vi "Get X Voltage.vi"(8 "error in (no error)":errorcluster, 11 "hdl in":i32) -> (0 "error out":errorcluster, 2 "Get x Voltage(V)":dbl, 3 "hdl":i32)   [LabVIEW 2011, in "Thorlabs_MDT69xB.lvlib"]
doc: "Reads and returns the X axis output voltage."
uses:
  <instrlib>/Thorlabs_MDT69xB/Thorlabs_MDT69xB.lvlib
  <instrlib>/Thorlabs_MDT69xB/Data/MDT_COMMAND_LIB_win32.dll
  <instrlib>/Thorlabs_MDT69xB/Data/MDT_COMMAND_LIB_x64.dll
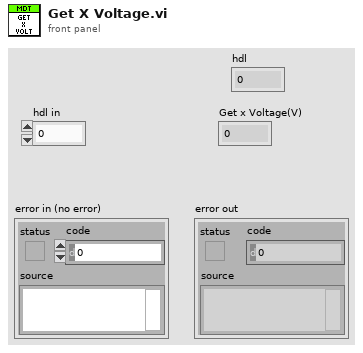
[diagram p1: front panel]
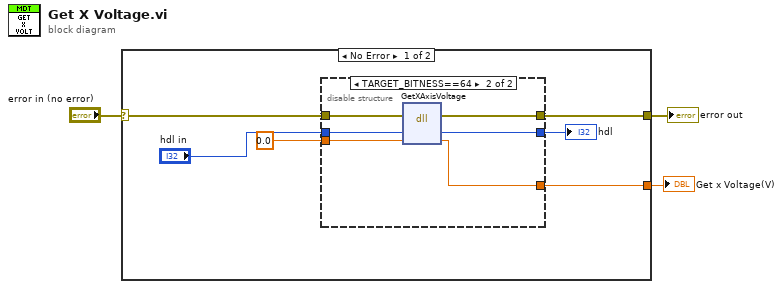
[diagram p0: block diagram]
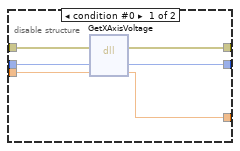
[diagram p2: hidden frame]
diagram:
  n1 = case shown="No Error" "error in (no error)" {
    selector: "error in (no error)" -> [w9 w22]
    tunnel: [w5 w22] -> w2
    tunnel: [w6 _] -> w1
    frame No Error {
      n2 = disable-structure shown="TARGET_BITNESS==64" {
        disable-tunnel: w9 -> [w15 w21]
        disable-tunnel: "hdl in" -> [w14 w20]
        disable-tunnel: 0.0 ("voltage") -> [w13 w19]
        disable-tunnel: [w12 w18] -> w6
        disable-tunnel: [w11 w17] -> w5
        disable-tunnel: [w10 w16] -> w4
        frame condition #0 {
          n3 = dll-call lib="C:/Program Files (x86)/National Instruments/LabVIEW 2011/instr.lib/Thorlabs_MDT69xB/Data/MDT_COMMAND_LIB_win32.dll" fn="GetXAxisVoltage"(error in=w15, "hdl"=w14, "voltage"=w13) -> (error out=w11:errorcluster, "hdl"=w10:i32, "voltage"=w12:dbl)  [unwired: 3 in, 1 out]
        }
        frame condition #1 (active) {
          n4 = dll-call lib="C:/Program Files/National Instruments/LabVIEW 2011/instr.lib/Thorlabs_MDT69xB/Data/MDT_COMMAND_LIB_x64.dll" fn="GetXAxisVoltage"(error in=w21, "hdl"=w20, "voltage"=w19) -> (error out=w17:errorcluster, "hdl"=w16:i32, "voltage"=w18:dbl)  [unwired: 3 in, 1 out]
        }
      }
      "hdl" <- w4
    }
    frame Error {
    }
  }
  "error out" <- w2
  "Get x Voltage(V)" <- w1
